vi "getDeltaFromRobotModel.vi"(11 "robotModel":dbl[][](array[numeric])) -> (3 "delta":dbl)   [LabVIEW 2021, in "Game.lvclass"]
uses:
  Game.lvclass
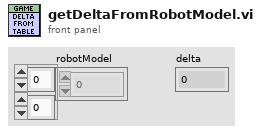
[diagram p1: front panel]
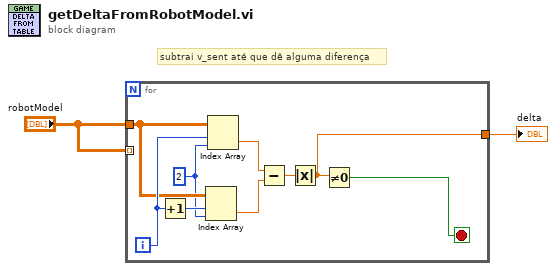
[diagram p0: block diagram]
diagram:
  # "subtrai v_sent até que dê alguma diferença"
  n1 = for {
    tunnel: "robotModel" -> [_] mode=indexing
    tunnel: "robotModel" -> [w9]
    tunnel: [w3] -> w2
    i -> [w10]
    stop <- w4 stop-if-true
    w8 = 2 ("index")
    n2 = Increment(x=w10) -> (x+1=w11:i32)
    n3 = Index Array(array=w9, index (row)=w11, index (col)=w8) -> (element=w6:dbl)
    n4 = Index Array(array=w9, index (row)=w10, index (col)=w8) -> (element=w7:dbl)
    n5 = Subtract(x=w7, y=w6) -> (x-y=w5:dbl)
    n6 = Absolute Value(x=w5) -> (abs(x)=w3:dbl)
    n7 = Not Equal To 0?(x=w3) -> (x != 0?=w4:bool)
  }
  "delta" <- w2
